vi "Untitled 2.vi"(1 "Action(GET)":enum16{"GET", "SET"}(ring), 7 "E&S Message in":T1, 11 "error in (no error)":errorcluster) -> (8 "E&S Message out":T1, 15 "error out":errorcluster)   [LabVIEW 2011]
uses:
  emi Lib/System 01/0 - General/S&E reporting/Private/_emi_ S&E Message type.ctl
  emi Lib/System 01/0 - General/S&E reporting/Private/_emi_ S&E Message.ctl
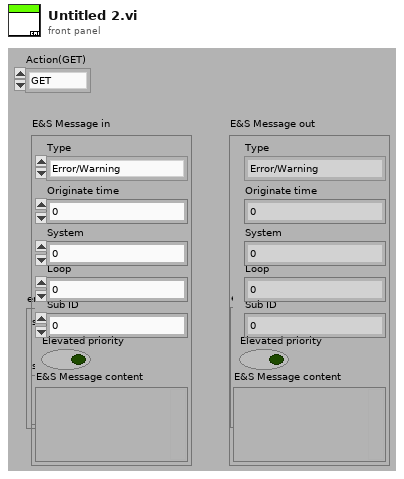
[diagram p1: front panel]
types:
  T1 = typedef "_emi_ S&E Message.ctl" = cluster{"Type":T2, "Originate time":dbl, "System":u8, "Loop":u16, "Sub ID":u16, "Elevated priority":bool, "E&S Message content":variant}
  T2 = typedef "_emi_ S&E Message type.ctl" = enum16{"Error/Warning", "Note", "Debug", "Event", "Alarm Analog", "Alarm Digital", "Annotation"}
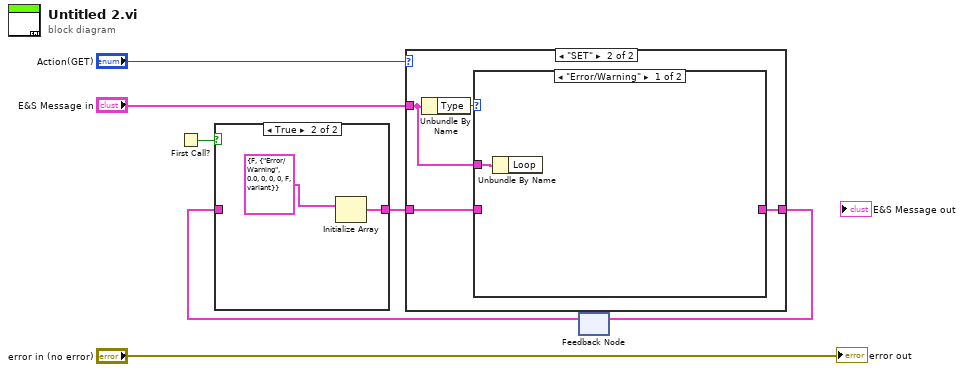
[diagram p0: block diagram]
diagram:
  n1 = First Call?() -> (First Call?: T/F=w4:bool)
  n2 = feedback #1() -> (w5:cluster{"Error":bool, "E&S Message":T1}[])  [unwired: 1 in]
  n3 = case shown="True" w4 {
    tunnel: w5 -> [w8 _]
    tunnel: [w8 w10] -> w2
    frame False {
    }
    frame True {
      n4 = Initialize Array(cluster{"Error":bool, "E&S Message":T1} {"Error"=FALSE, "E&S Message"={"Type"=enum."Error/Warning", "Originate time"=0.0, "System"=0, "Loop"=0, "Sub ID"=0, "Elevated priority"=FALSE, "E&S Message content"=variant}}) -> (w10:cluster{"Error":bool, "E&S Message":T1}[])  [unwired: 1 in]
    }
  }
  n5 = case shown="\"SET\"" "Action(GET)" {
    tunnel: [w11 w14] -> w3
    tunnel: w2 -> [w11 w13]
    tunnel: "E&S Message in" -> [_ w12]
    frame "GET", Default {
    }
    frame "SET" {
      n6 = Unbundle By Name(w12) -> ("Type"=w15:T2)
      n7 = case shown="\"Error/Warning\"" w15 {
        tunnel: [_ w17] -> w14
        tunnel: w13 -> [_ w17]
        tunnel: w12 -> [w16 _]
        frame "Error/Warning" {
          n8 = Unbundle By Name(w16) -> ()  [unwired: 1 out]
        }
        frame "Note", Default {
        }
      }
    }
  }
  n9 = feedback-in #1(w3) -> ()
  "error out" <- "error in (no error)"
